vi "connect to data network stream.vi"(10 "Data in":T1={"Parameters"={"FPGA Ref"=refnum, "data stream"={"data writer name"="error writer", "NS write buffer size"=16, "NS Buffer length"=0}, "FIFO Depth"=0, "Channel controls"={"FIFO channel count"=0, "active indices"=[], "active channels"=0, "channelScaling"=[], "scanivalveCount"=0, "channels"=[]}, "safetyChannels"={"oilP"=0, "airP"=0, "water"=0, "channelLimits"=[]}, "speedChannel"=0, "maxSpeedLimit"=0.0, "Torque"={"fixedOffset"=0.0, "filter"=FALSE, "fallingEdge"=FALSE, "swapEncoders"=FALSE}}, "Variables"={"Intermediary buffer"=[], "buffer position"=0, "write loop counter"=0, "NS write trigger"=0, "NS Connection status"=FALSE, "waiting for NS"=FALSE, "labAmbient"={"pressure"=0.0, "temperature"=0.0}, "scanivalvePorts"=[], "scanivalvePressures"=[], "data stream"="", "activeChannelLimitIndex"=[], "runningSpeedLimit"=0.0, "speedChannelIndex"=0, "Interlocks"={"gearboxOil"=FALSE, "bearingOil"=FALSE, "gearboxAir"=FALSE}, "interlockChannels"={"gearboxOil"=0, "bearingOil"=0, "air"=0}, "limitStates"=[]}}, 11 "RT Queues":T8) -> (3 "Data out":T1={"Parameters"={"FPGA Ref"=refnum, "data stream"={"data writer name"="error writer", "NS write buffer size"=16, "NS Buffer length"=0}, "FIFO Depth"=0, "Channel controls"={"FIFO channel count"=0, "active indices"=[], "active channels"=0, "channelScaling"=[], "scanivalveCount"=0, "channels"=[]}, "safetyChannels"={"oilP"=0, "airP"=0, "water"=0, "channelLimits"=[]}, "speedChannel"=0, "maxSpeedLimit"=0.0, "Torque"={"fixedOffset"=0.0, "filter"=FALSE, "fallingEdge"=FALSE, "swapEncoders"=FALSE}}, "Variables"={"Intermediary buffer"=[], "buffer position"=0, "write loop counter"=0, "NS write trigger"=0, "NS Connection status"=FALSE, "waiting for NS"=FALSE, "labAmbient"={"pressure"=0.0, "temperature"=0.0}, "scanivalvePorts"=[], "scanivalvePressures"=[], "data stream"="", "activeChannelLimitIndex"=[], "runningSpeedLimit"=0.0, "speedChannelIndex"=0, "Interlocks"={"gearboxOil"=FALSE, "bearingOil"=FALSE, "gearboxAir"=FALSE}, "interlockChannels"={"gearboxOil"=0, "bearingOil"=0, "air"=0}, "limitStates"=[]}})   [LabVIEW 2018]
uses:
  Type Defs/Queues cluster.ctl
  ICL-LabVIEW_General/Message Scheduler/message scheduler.lvclass
  Type Defs/Data processing loop data.ctl
  Type Defs/FPGA reference.ctl
  PC/type defs/channelControl.ctl
  Type Defs/channelScalingTypes.ctl
  Type Defs/scalingMethods.ctl
  ICL-LabVIEW_General/data channels/parent class/Data Channel.lvclass
  PC/type defs/channelLimitControl.ctl
  PC/type defs/limitActions.ctl
  <resource>/objmgr/ni.dex.rc
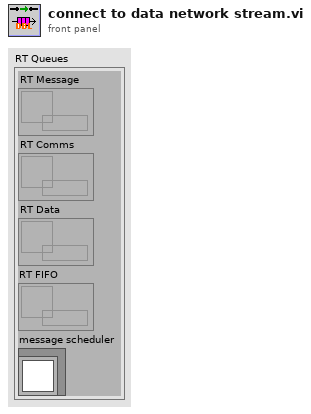
[diagram p1: front panel]
types:
  T1 = typedef "Data processing loop data.ctl" = cluster{"Parameters":cluster{"FPGA Ref":T2, "data stream":cluster{"data writer name":string, "NS write buffer size":i32, "NS Buffer length":u32}, "FIFO Depth":u32, "Channel controls":cluster{"FIFO channel count":i32, "active indices":i16[], "active channels":i32, "channelScaling":T3[], "scanivalveCount":i32, "channels":refnum<class "Data Channel.lvclass">[]}, "safetyChannels":cluster{"oilP":u16, "airP":u16, "water":u16, "channelLimits":T6[]}, "speedChannel":i32, "maxSpeedLimit":dbl, "Torque":cluster{"fixedOffset":dbl, "filter":bool, "fallingEdge":bool, "swapEncoders":bool}}, "Variables":cluster{"Intermediary buffer":dbl[][], "buffer position":u32, "write loop counter":u16, "NS write trigger":u32, "NS Connection status":bool, "waiting for NS":bool, "labAmbient":cluster{"pressure":dbl, "temperature":dbl}, "scanivalvePorts":u16[], "scanivalvePressures":dbl[], "data stream":refnum<k21>, "activeChannelLimitIndex":u16[], "runningSpeedLimit":dbl, "speedChannelIndex":i32, "Interlocks":cluster{"gearboxOil":bool, "bearingOil":bool, "gearboxAir":bool}, "interlockChannels":cluster{"gearboxOil":i32, "bearingOil":i32, "air":i32}, "limitStates":cluster{"warn":bool, "alarm":bool}[]}}
  T2 = typedef "FPGA reference.ctl" = refnum<k20>
  T3 = typedef "channelControl.ctl" = cluster{"index":u16, "active":bool, "channelType":T4, "module":u16, "terminal":u16, "channelName":string, "scalingMethod":T5, "scalingParameters":dbl[], "scaledUnits":string, "tempOffset":dbl}
  T4 = typedef "channelScalingTypes.ctl" = enum16{"calculation", "measurement", "scanivalve", "output", "digital"}
  T5 = typedef "scalingMethods.ctl" = enum16{"none", "linear", "thermocouple", "polynomial", "encoder", "RTD"}
  T6 = typedef "channelLimitControl.ctl" = cluster{"channelID":u16, "Enabled":bool, "warnValue":dbl, "limitValue":dbl, "Invert":bool, "limitAction":T7}
  T7 = typedef "limitActions.ctl" = enum16{"stop", "shutdown", "ignore"}
  T8 = typedef "Queues cluster.ctl" = cluster{"RT Message":refnum<queue>, "RT Comms":refnum<queue>, "RT Data":refnum<queue>, "RT FIFO":refnum<queue>, "message scheduler":refnum<class "message scheduler.lvclass">}
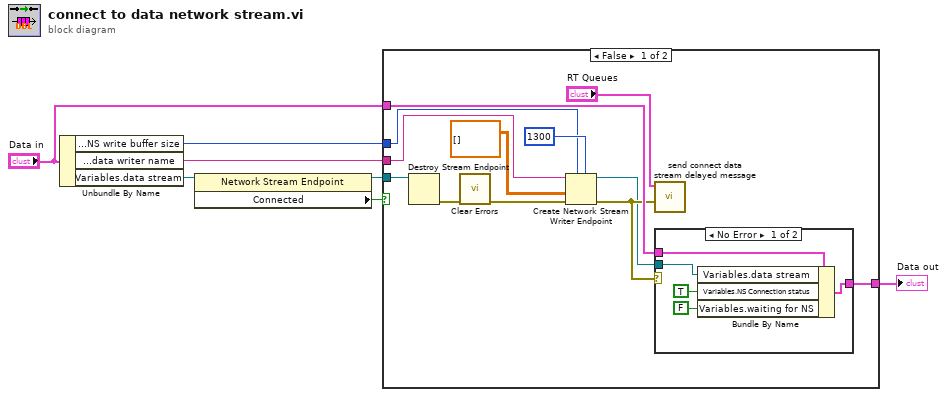
[diagram p0: block diagram]
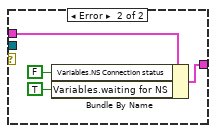
[diagram p2: hidden frame]
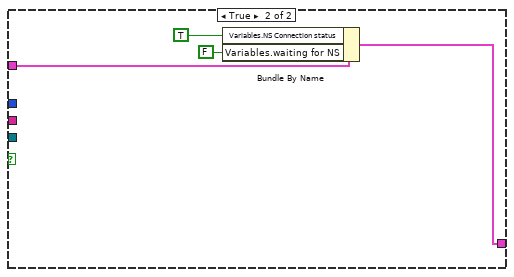
[diagram p3: hidden frame]
diagram:
  n1 = Unbundle By Name("Data in") -> ("Parameters.data stream.NS write buffer size"=w6:i32, "Parameters.data stream.data writer name"=w5:string, "Variables.data stream"=w3:refnum<k21>)
  n2 = property class="Network Stream Endpoint"(reference=w3) -> (reference out=w1:refnum<k21>, "Connected"=w2:bool)  [unwired: 1 in, 1 out]
  n3 = case shown="False" w2 {
    tunnel: [w18 w31] -> w7
    tunnel: w6 -> [w15 _]
    tunnel: w5 -> [w14 _]
    tunnel: "Data in" -> [w13 w32]
    tunnel: w1 -> [w12 _]
    frame False {
      n4 = Destroy Stream Endpoint(11:w12) -> (0:w11:errorcluster)  [unwired: 1 in]
      n5 = call <vilib>:"Clear Errors.vi"("error in (no error)"=w11) -> ("error out"=w10:errorcluster)  [unwired: 5 in, 1 out]
      n6 = Create Network Stream Writer Endpoint(5:1300 ("timeout in ms (-1)"), 7:w15, 8:w10, 9:dbl[][] [], 11:w14) -> (0:w9:errorcluster, 3:w8:refnum<k21>)  [unwired: 2 in]
      n7 = call "send connect data stream delayed message.vi"("error"=w9, "RT Queues"="RT Queues") -> ()  [unwired: 10 in]
      n8 = case shown="No Error" w9 {
        tunnel: w8 -> [w24 _]
        tunnel: [w23 w28] -> w18
        tunnel: w13 -> [w22 w27]
        frame No Error {
          n9 = Bundle By Name(cluster=w22, "Variables.data stream"=w24, "Variables.NS Connection status"=TRUE, "Variables.waiting for NS"=FALSE) -> (w23:T1)
        }
        frame Error {
          n10 = Bundle By Name(cluster=w27, "Variables.NS Connection status"=FALSE, "Variables.waiting for NS"=TRUE) -> (w28:T1)
        }
      }
    }
    frame True {
      n11 = Bundle By Name(cluster=w32, "Variables.NS Connection status"=TRUE, "Variables.waiting for NS"=FALSE) -> (w31:T1)
    }
  }
  "Data out" <- w7
